vi "ScanBeam_Config.vi"() -> ()   [LabVIEW 2016]
panel:
  in  "Boolean 4":bool
  in  "Beam Rotation Array":T1(array[cluster])=[{"TX1"=1, "TX2"=1, "TX3"=1, "TX4"=1, "TXx3"=1, "TXx4"=1, "RX1"=2, "RX2"=2, "RX3"=2, "RX4"=2, "RXx3"=2, "RXx4"=2}, {"TX1"=15, "TX2"=15, "TX3"=15, "TX4"=15, "TXx3"=15, "TXx4"=15, "RX1"=16, "RX2"=16, "RX3"=16, "RX4"=16, "RXx3"=16, "RXx4"=16}, {"TX1"=19, "TX2"=19, "TX3"=19, "TX4"=19, "TXx3"=19, "TXx4"=19, "RX1"=20, "RX2"=20, "RX3"=20, "RX4"=20, "RXx3"=20, "RXx4"=20}]
  # "Rotation"
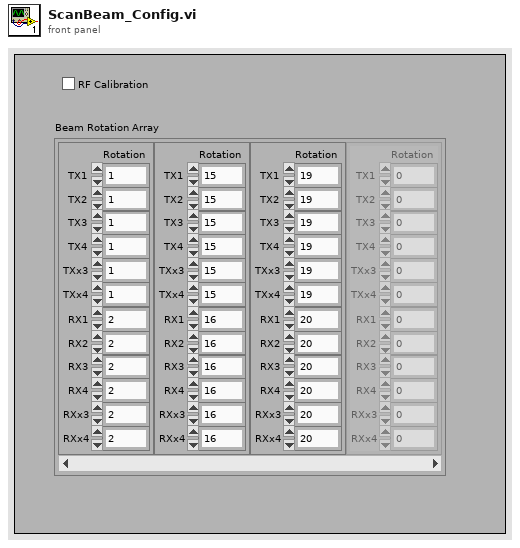
[diagram p1: front panel]
types:
  T1 = cluster{"TX1":i32, "TX2":i32, "TX3":i32, "TX4":i32, "TXx3":i32, "TXx4":i32, "RX1":i32, "RX2":i32, "RX3":i32, "RX4":i32, "RXx3":i32, "RXx4":i32}[]
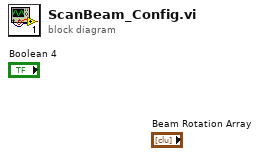
[diagram p0: block diagram]
diagram:
